vi "position_zu_boundig_rectangle_mit_farbe.vi"(6 "y":sgl, 7 "Color":u32, 9 "größe in":sgl, 10 "x":sgl, 11 "Refnum in":T1) -> (3 "Refnum out":T1)   [LabVIEW 2014]
uses:
  <vilib>/vision/Image Controls.llb/IMAQ Image.ctl
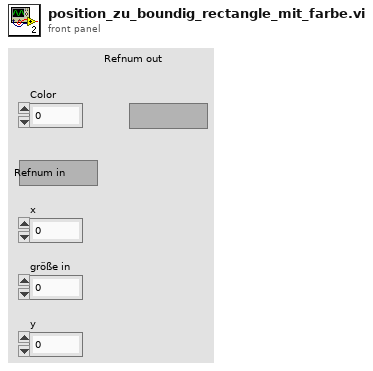
[diagram p1: front panel]
types:
  T1 = typedef "IMAQ Image.ctl" = refnum<image>
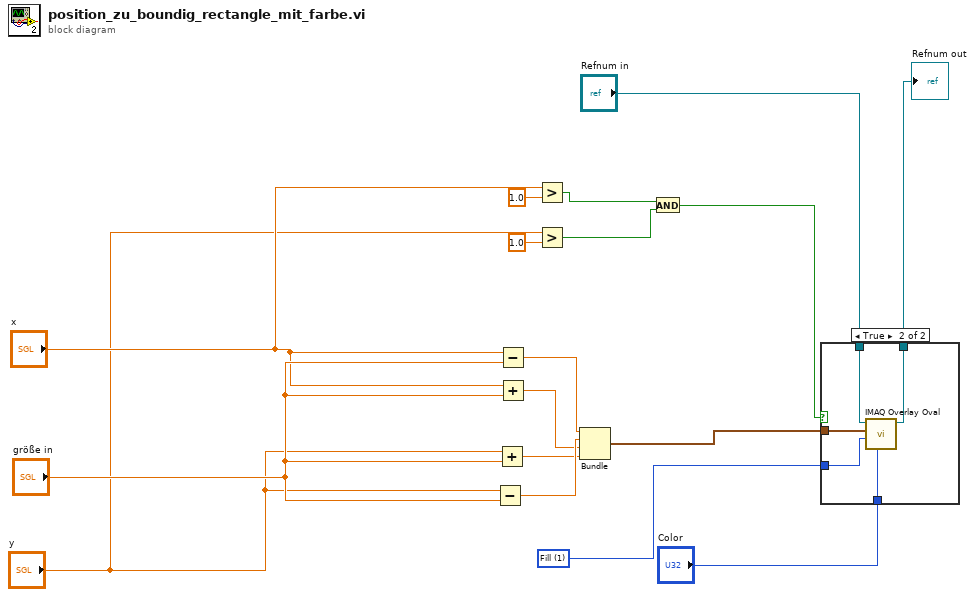
[diagram p0: block diagram]
diagram:
  w9 = u32 1 items=["Frame", "Fill"] ("Drawing Mode (Frame)")
  n1 = Subtract(x="y", y="größe in") -> (x-y=w14:sgl)
  n2 = Add(x="y", y="größe in") -> (x+y=w12:sgl)
  n3 = Subtract(x="x", y="größe in") -> (x-y=w15:sgl)
  n4 = Add(x="x", y="größe in") -> (x+y=w13:sgl)
  n5 = Greater?(x="x", y=sgl 1.0) -> (0:w3:bool)
  n6 = Greater?(x="y", y=sgl 1.0) -> (0:w2:bool)
  n7 = Bundle(w15, w14, w13, w12) -> (w11:cluster{sgl, sgl, sgl, sgl})  [unwired: 1 in]
  n8 = And(x=w3, y=w2) -> (x .and. y?=w1:bool)
  n9 = case shown="True" w1 {
    tunnel: [w18 w23] -> w17
    tunnel: "Refnum in" -> [w18 w22]
    tunnel: w11 -> [_ w21]
    tunnel: "Color" -> [_ w20]
    tunnel: w9 -> [_ w19]
    frame False {
    }
    frame True {
      n10 = call "IMAQ Overlay Oval"("Color"=w20, "Drawing Mode (Frame)"=w19, "Bounding Rectangle"=w21, "Image"=w22) -> ("Image Out"=w23:T1)  [unwired: 6 in, 1 out]
    }
  }
  "Refnum out" <- w17
